vi "待机状态数据存储写入和切换量程(子VI).vi"   [LabVIEW 2016, in "斯坦道CODMn.lvlib"]
uses:
  <vilib>/ptbypt/NI_PtbyPt.lvlib
types:
  T1 = cluster{"时间":timestamp, "测量模式":string, "数据类型":string, "检测值":sgl, "单位":string, "数据标识":string, "因子编码":string, "标样参考值":sgl, "ORP-A":sgl, "ORP-B":sgl, "ORP-K":sgl, "COD滴定值":sgl, "高锰酸钾滴定数":sgl, "温度":sgl, "量程":sgl, "LastTime":timestamp}
  T2 = cluster{"因子编码":u32, "单位":u16, "标样参考值":sgl, "水样数据时间":timestamp, "水样实测值":sgl, "水样数据标识":string, "标样数据时间":timestamp, "标样实测值":sgl, "标样数据标识":string, "空白数据时间":timestamp, "空白实测值":sgl, "空白数据标识":string, "零点核查数据时间":timestamp, "零点核查实测值":sgl, "零点核查数据标识":string, "跨度核查数据时间":timestamp, "跨度核查实测值":sgl, "跨度核查数据标识":string, "加标回收数据时间":timestamp, "加标回收实测值":sgl, "加标回收数据标识":string, "平行样数据时间":timestamp, "平行样实测值":sgl, "平行样数据标识":string}
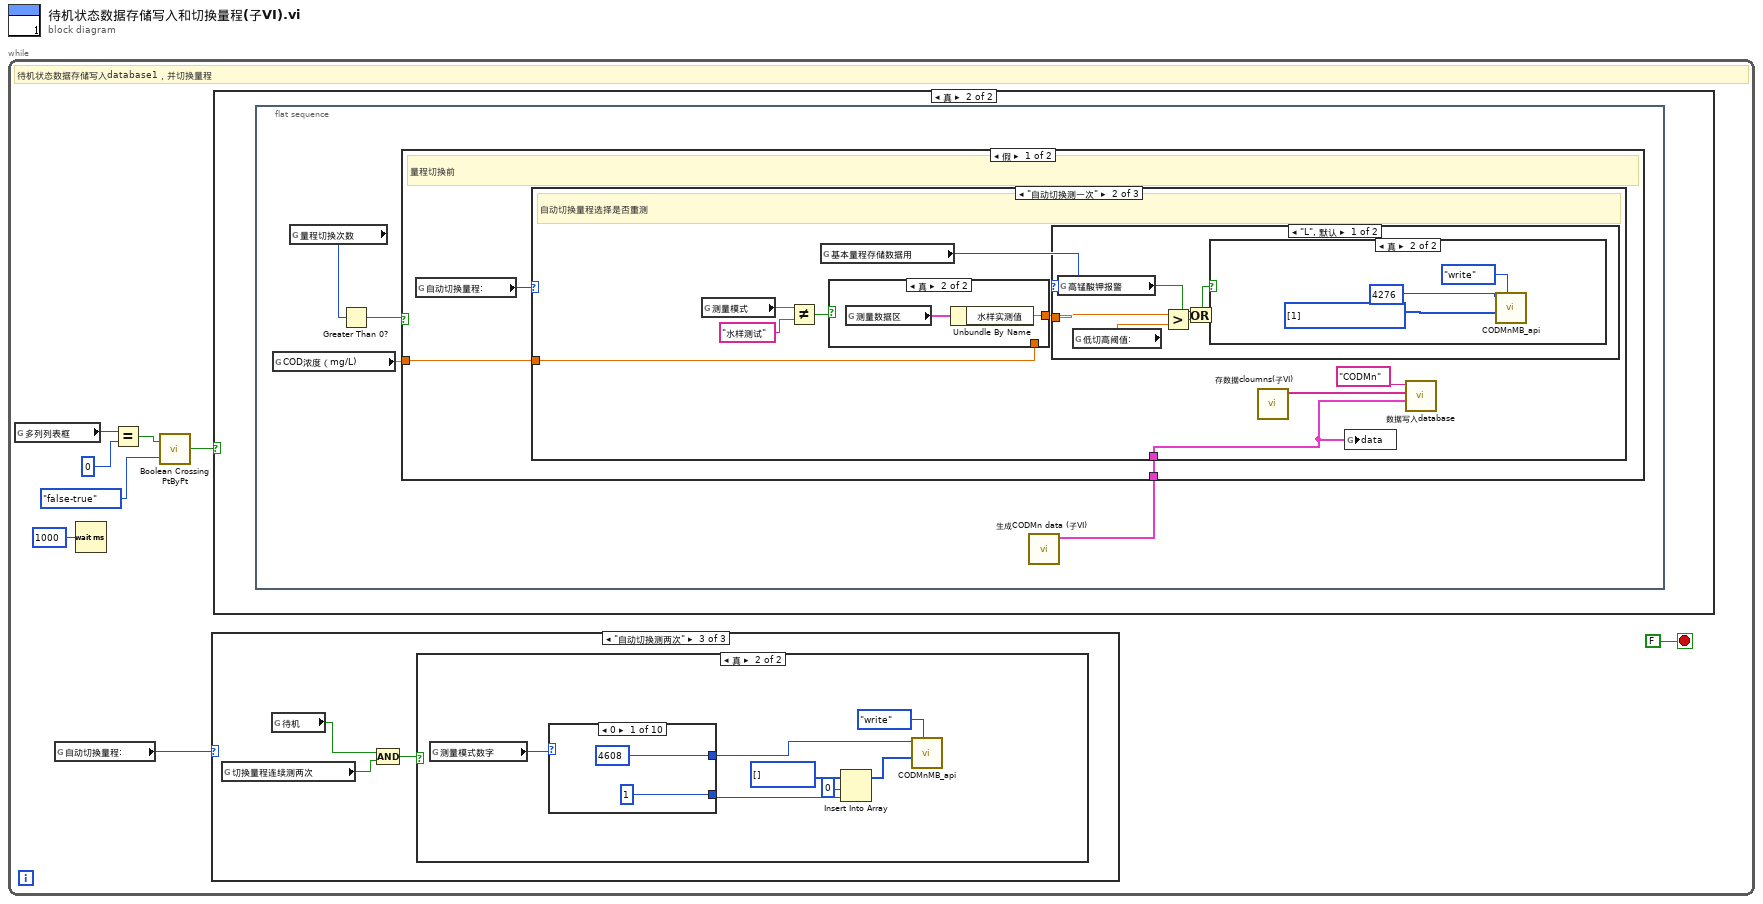
[diagram p0: block diagram]
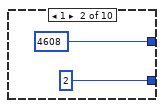
[diagram p5: hidden frame]
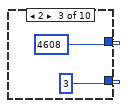
[diagram p6: hidden frame]
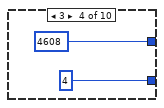
[diagram p7: hidden frame]
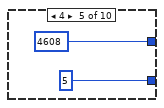
[diagram p8: hidden frame]
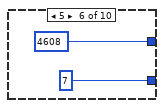
[diagram p9: hidden frame]
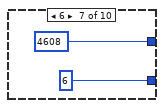
[diagram p10: hidden frame]
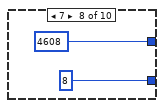
[diagram p11: hidden frame]
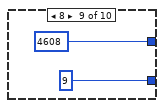
[diagram p12: hidden frame]
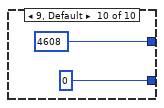
[diagram p13: hidden frame]
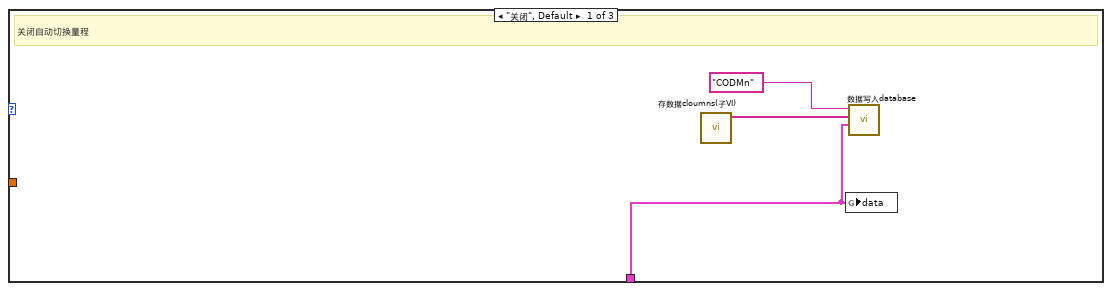
[diagram p15: hidden frame]
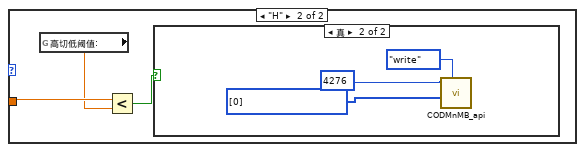
[diagram p17: hidden frame]
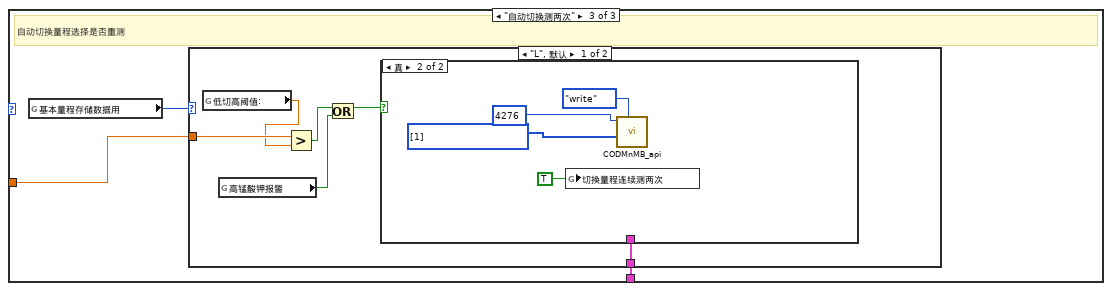
[diagram p20: hidden frame]
diagram:
  n1 = while {
    stop <- FALSE stop-if-true
    # "待机状态数据存储写入database1，并切换量程"
    n2 = global read "运行时序全局变量.vi" "多列列表框"() -> (w2:i32)
    n3 = global read "CODMn断电保存全局变量.vi" "自动切换量程:"() -> (w1:enum16{"关闭", "自动切换测一次", "自动切换测两次"})
    n4 = Wait (ms)(milliseconds to wait=u32 1000 ("等待时间（毫秒）")) -> ()  [unwired: 1 out]
    n5 = Equal?(x=w2, y=0) -> (x = y?=w5:bool)
    n6 = call <vilib>:"Boolean Crossing PtByPt.vi"("direction"=enum16{"either", "false-true", "true-false"}."false-true", "input"=w5) -> ("crossing"=w3:bool)  [unwired: 1 in]
    n7 = case shown="\"自动切换测两次\"" w1 {
      frame "关闭", Default {
      }
      frame "自动切换测一次" {
      }
      frame "自动切换测两次" {
        n8 = global read "COD内部交互全局.vi" "切换量程连续测两次"() -> (w10:bool)
        n9 = global read "COD内部交互全局.vi" "待机"() -> (w9:bool)
        n10 = Compound Arithmetic op=AND ("复合运算")(w9, w10) -> (w11:bool)
        n11 = case shown="真" w11 {
          frame False {
          }
          frame True {
            n12 = global read "COD内部交互全局.vi" "测量模式数字"() -> (w12:i32)
            n13 = case shown="0" w12 {
              tunnel: [u16 4608 ("address") u16 4608 ("address") u16 4608 ("address") u16 4608 ("address") u16 4608 ("address") u16 4608 ("address") u16 4608 ("address") u16 4608 ("address") u16 4608 ("address") u16 4608 ("address")] -> w13
              tunnel: [u16 1 ("address") u16 2 ("address") u16 3 ("address") u16 4 ("address") u16 5 ("address") u16 7 ("address") u16 6 ("address") u16 8 ("address") u16 9 ("address") u16 0 ("address")] -> w18
              frame 0 {
              }
              frame 1 {
              }
              frame 2 {
              }
              frame 3 {
              }
              frame 4 {
              }
              frame 5 {
              }
              frame 6 {
              }
              frame 7 {
              }
              frame 8 {
              }
              frame 9, Default {
              }
            }
            n14 = Insert Into Array(array=u16[] [] ("values"), index=0 ("索引"), new element=w18) -> (w14:u16[])
            n15 = call "CODMnMB_api.vi"("STEP"=enum16{"open", "read", "write", "close"}."write", "values"=w14, "starting address"=w13) -> ()  [unwired: 6 in, 3 out]
          }
        }
      }
    }
    n16 = case shown="真" w3 {
      frame False {
      }
      frame True {
        n17 = flat-sequence {
          frame #0 {
            n18 = global read "COD浓度全局变量.vi" "COD浓度（mg/L)"() -> (w40:dbl)
            n19 = global read "COD内部交互全局.vi" "量程切换次数"() -> (w39:u8)
            n20 = Greater Than 0?(x=w39) -> (x > 0?=w41:bool)
            n21 = call "生成CODMn data (子VI).vi"() -> ("data"=w42:T1)  [unwired: 11 in]
            n22 = case shown="假" w41 {
              tunnel: w42 -> [w45 w103]
              tunnel: w40 -> [w44 _]
              frame False {
                # "量程切换前"
                n23 = global read "CODMn断电保存全局变量.vi" "自动切换量程:"() -> (w43:enum16{"关闭", "自动切换测一次", "自动切换测两次"})
                n24 = case shown="\"自动切换测一次\"" w43 {
                  tunnel: w45 -> [w46 w51 w77]
                  tunnel: w44 -> [_ w50 w76]
                  frame "关闭", Default {
                    # "关闭自动切换量程"
                    n25 = call "存数据cloumns(子VI).vi"() -> ("数组"=w48:string[])  [unwired: 11 in]
                    n26 = global write "COD内部交互全局.vi" "data"(w46) -> ()
                    n27 = call "数据写入database.vi"("data"=w46, "columns"=w48, "table"="CODMn") -> ()  [unwired: 8 in, 1 out]
                  }
                  frame "自动切换测一次" {
                    # "自动切换量程选择是否重测"
                    n28 = global read "COD测量模式全局.vi" "测量模式"() -> (w57:string)
                    n29 = Not Equal?(x=w57, y="水样测试") -> (x != y?=w55:bool)
                    n30 = global read "COD内部交互全局.vi" "基本量程存储数据用"() -> (w49:enum16{"L", "H"})
                    n31 = case shown="真" w55 {
                      tunnel: [w72 w73] -> w54
                      tunnel: w50 -> [w72 _]
                      frame False {
                      }
                      frame True {
                        n32 = global read "CODMn断电保存全局变量.vi" "测量数据区"() -> (w74:T2)
                        n33 = Unbundle By Name(w74) -> ("水样实测值"=w73:sgl)
                      }
                    }
                    n34 = case shown="\"L\", 默认" w49 {
                      tunnel: w54 -> [w61 w67]
                      frame "L", Default {
                        n35 = global read "COD内部交互全局.vi" "高锰酸钾报警"() -> (w58:bool)
                        n36 = global read "CODMn断电保存全局变量.vi" "低切高阈值:"() -> (w59:dbl)
                        n37 = Greater?(x=w61, y=w59) -> (0:w62:bool)
                        n38 = Or(x=w58, y=w62) -> (x .or. y?=w60:bool)
                        n39 = case shown="真" w60 {
                          frame False {
                          }
                          frame True {
                            n40 = call "CODMnMB_api.vi"("STEP"=enum16{"open", "read", "write", "close"}."write", "values"=u16[] [1], "starting address"=u16 4276) -> ()  [unwired: 6 in, 3 out]
                          }
                        }
                      }
                      frame "H" {
                        n41 = global read "CODMn断电保存全局变量.vi" "高切低阈值:"() -> (w66:dbl)
                        n42 = Less?(x=w67, y=w66) -> (x < y?=w68:bool)
                        n43 = case shown="真" w68 {
                          frame False {
                          }
                          frame True {
                            n44 = call "CODMnMB_api.vi"("STEP"=enum16{"open", "read", "write", "close"}."write", "values"=u16[] [0], "starting address"=u16 4276) -> ()  [unwired: 6 in, 3 out]
                          }
                        }
                      }
                    }
                    n45 = call "存数据cloumns(子VI).vi"() -> ("数组"=w53:string[])  [unwired: 11 in]
                    n46 = global write "COD内部交互全局.vi" "data"(w51) -> ()
                    n47 = call "数据写入database.vi"("data"=w51, "columns"=w53, "table"="CODMn") -> ()  [unwired: 8 in, 1 out]
                  }
                  frame "自动切换测两次" {
                    # "自动切换量程选择是否重测"
                    n48 = global read "COD内部交互全局.vi" "基本量程存储数据用"() -> (w75:enum16{"L", "H"})
                    n49 = case shown="\"L\", 默认" w75 {
                      tunnel: w76 -> [w82 w93]
                      tunnel: w77 -> [w81 w92]
                      frame "L", Default {
                        n50 = global read "CODMn断电保存全局变量.vi" "低切高阈值:"() -> (w79:dbl)
                        n51 = global read "COD内部交互全局.vi" "高锰酸钾报警"() -> (w78:bool)
                        n52 = Greater?(x=w82, y=w79) -> (0:w83:bool)
                        n53 = Or(x=w83, y=w78) -> (x .or. y?=w80:bool)
                        n54 = case shown="真" w80 {
                          tunnel: w81 -> [w84 _]
                          frame False {
                            n55 = call "存数据cloumns(子VI).vi"() -> ("数组"=w86:string[])  [unwired: 11 in]
                            n56 = global write "COD内部交互全局.vi" "data"(w84) -> ()
                            n57 = call "数据写入database.vi"("data"=w84, "columns"=w86, "table"="CODMn") -> ()  [unwired: 8 in, 1 out]
                          }
                          frame True {
                            n58 = global write "COD内部交互全局.vi" "切换量程连续测两次"(TRUE ("切换量程连续测两次")) -> ()
                            n59 = call "CODMnMB_api.vi"("STEP"=enum16{"open", "read", "write", "close"}."write", "values"=u16[] [1], "starting address"=u16 4276) -> ()  [unwired: 6 in, 3 out]
                          }
                        }
                      }
                      frame "H" {
                        n60 = global read "CODMn断电保存全局变量.vi" "高切低阈值:"() -> (w91:dbl)
                        n61 = Less?(x=w93, y=w91) -> (x < y?=w94:bool)
                        n62 = case shown="真" w94 {
                          tunnel: w92 -> [w95 _]
                          frame False {
                            n63 = call "存数据cloumns(子VI).vi"() -> ("数组"=w97:string[])  [unwired: 11 in]
                            n64 = global write "COD内部交互全局.vi" "data"(w95) -> ()
                            n65 = call "数据写入database.vi"("data"=w95, "columns"=w97, "table"="CODMn") -> ()  [unwired: 8 in, 1 out]
                          }
                          frame True {
                            # "重测第一次不存数据"
                            n66 = call "CODMnMB_api.vi"("STEP"=enum16{"open", "read", "write", "close"}."write", "values"=u16[] [0], "starting address"=u16 4276) -> ()  [unwired: 6 in, 3 out]
                            n67 = global write "COD内部交互全局.vi" "切换量程连续测两次"(TRUE ("切换量程连续测两次")) -> ()
                          }
                        }
                      }
                    }
                  }
                }
              }
              frame True {
                # "防止无限切量程"
                n68 = global write "COD内部交互全局.vi" "量程切换次数"(u8 0 ("量程切换次数")) -> ()
                n69 = call "存数据cloumns(子VI).vi"() -> ("数组"=w105:string[])  [unwired: 11 in]
                n70 = call "数据写入database.vi"("data"=w103, "columns"=w105, "table"="CODMn") -> ()  [unwired: 8 in, 1 out]
                n71 = global write "COD内部交互全局.vi" "data"(w103) -> ()
              }
            }
          }
        }
      }
    }
  }
